vi "Close-log.vi"(8 "error in (no error)":errorcluster, 11 "Errors in":T1) -> (0 "error out":errorcluster, 3 "Errors out":T1)   [LabVIEW 2013, in "Error-handling.lvlib" / "Errors.lvclass"]
uses:
  Errors.lvclass
  Object-reference.ctl
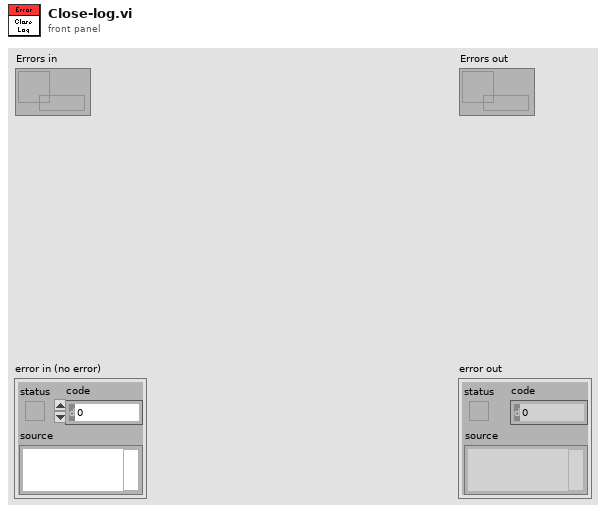
[diagram p1: front panel]
types:
  T1 = typedef "Error-handling.lvlib/Errors.lvclass/Object-reference.ctl" = refnum<data-value>
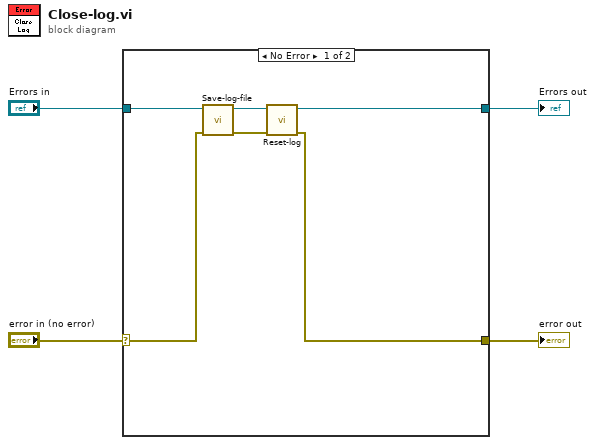
[diagram p0: block diagram]
diagram:
  n1 = case shown="No Error" "error in (no error)" {
    selector: "error in (no error)" -> [w7 w12]
    tunnel: [w5 w12] -> w3
    tunnel: [w8 w11] -> w1
    tunnel: "Errors in" -> [w10 w11]
    frame No Error {
      n2 = call "Save-log-file.vi"("error in (no error)"=w7, "Errors in"=w10) -> ("error out"=w6:errorcluster, "Errors out"=w9:T1)  [unwired: 8 in]
      n3 = call "Reset-log.vi"("error in (no error)"=w6, "Errors in"=w9) -> ("error out"=w5:errorcluster, "Errors out"=w8:T1)  [unwired: 8 in]
    }
    frame Error {
    }
  }
  "error out" <- w3
  "Errors out" <- w1
